vi "JTAG Panel.vi"() -> ()   [LabVIEW 2009]
panel:
  in  "Function":u16(ring) items=["READ_IO_VARS"=0, "PORT_OUT"=1, "PORT_SEL"=2, "PORT_REN"=3, "PORT_IN"=4, "PORT_DIR"=5, "SET_LCM"=6, "PWR_WRITE_SINGLE"=12, "PWR_READ_SINGLE"=13, "PWR_WRITE_MASK"=16, "PWR_WRITE_TRIM_DEFAULTS"=17, "STIM_POWER_UP"=20, "STIM_POWER_DN"=21, "STIM_WRITE_SINGLE"=22, "STIM_READ_SINGLE"=23, "STIM_WRITE_BLOCK"=24, "STIM_READ_BLOCK"=25, "STIM_WRITE_MASK"=26, "MICS_POWER_UP"=30, "MICS_POWER_DN"=31, "MICS_WRITE_SINGLE"=32, "MICS_READ_SINGLE"=33, "MICS_WRITE_BLOCK"=34, "MICS_READ_BLOCK"=35, "MICS_WRITE_MASK"=36, "MEM_POWER_UP"=40, "MEM_POWER_DN"=41, "MEM_WRITE_SINGLE"=42, "MEM_READ_SINGLE"=43, "MEM_WRITE_BLOCK"=44, "MEM_READ_BLOCK"=45, "MEM_WRITE_MASK"=46, "MEM_WRITE_SR"=47, "MEM_READ_SR"=48, "MEM_WRITE_OPCODE"=49, "INIT_PORTS"=50, "INIT_COMMS"=60, "RELEASE_COMMS"=61, "INIT_VARS"=62, "DCO_1MHZ"=63, "DCO_8MHZ"=64, "STANDARD_STARTUP"=65, "SET_LCM"=66, "PLUTO_WRITE_TRIM_DEFAULTS"=67, "SATURN_DIG_STARTUP"=68, "SATURN_BBC_STARTUP"=69, "SATURN_BBC_SHUTDOWN"=70, "START_STIM_CLK"=80, "STOP_STIM_CLK"=81, "PULSE_STIM_CLK"=82, "PULSE_STIM_SCK"=83, "SINGLE_ADC12"=85, "SINGLE_ADC12_REPEAT"=86, "MULTI_ADC12"=87, "MULTI_ADC12_REPEAT"=88, "DISABLE_ADC12"=89, "TC_STIM_RAM_READ"=200, "TC_STIM_RAM_WRITE"=201, "TC_TIMING_TEST"=220]
  out "error out":errorcluster
  out "MD5 message-digest out":string
  out "Status":bool
  in  "MD5 message-digest in":string
  in  "Function":T1(ring)
  in  "File Path":path=path "C:/Documents and Settings/Operator/My Documents/workspace_2/Test_Firmware_V1/Release/Test_Firmware_V1.txt"
  in  "Do Program":bool
  out "error out 3":errorcluster
  out "ARG1-ARG7":u16[](array[numeric]) format="%04x"
  out "ARG 7":u16 format="%04x"
  in  "ARG 6":u16 format="%04x"
  in  "ARG 5":u16 format="%04x"
  in  "ARG 4":u16 format="%04x"
  in  "ARG 3":u16 format="%04x"
  in  "ARG 2":u16 format="%04x"
  in  "ARG 1":u16 format="%04x"
  in  "Quick Bit Function (Manual)":T2(ring)
  in  "Function":u16(ring)=3 items=["Power UP", "Power DN", "Write Single", "Read Single", "Write Block", "Read Block", "Write Masked", "Test Value"]
  in  "State (L)":bool
  in  "RESET TARGET":bool
  in  "START MCU ZERO":bool
  in  "START MCU":bool
  in  "Sync JTAG (STOP MCU)":bool
  out "Device Vcc":dbl
  out "error out":errorcluster
  out "Block Read Data":u16[](array[numeric]) format="%02x"
  out "Test Result":bool
  out "Read Value":u8 format="%02x"
  in  "Block Write Data":u8[](array[numeric]) format="%02x"
  in  "Blocksize":u16
  in  "Target":u16(ring) items=["Power ASIC", "Stim ASIC", "MICS Radio", "FRAM"]
  in  "Address":u16 format="%04x"
  in  "Value":u8 format="%02x"
  in  "Mask":u8 format="%02x"
  in  "SPI":bool
  in  "Buffer Address (Byte from Buffer)":u16=4352 format="%x"
  out "Byte OUT (Byte from Buffer)":u8 format="%x"
  in  "Byte from Buffer":bool
  in  "Buffer Address (Byte to Buffer)":u16=4352 format="%x"
  in  "Byte IN (Byte to Buffer)":u8
  in  "Byte to Buffer":bool
  in  "Block size (Buffer to RAM)":u16=18 format="%x"
  in  "Start address (Buffer to RAM)":u16=4352 format="%x"
  in  "Buffer to RAM":bool
  in  "Block size (RAM to Buffer)":u16=18 format="%x"
  in  "Start address (RAM to Buffer)":u16=4352 format="%x"
  in  "RAM to Buffer":bool
  in  "Power Target Device (Init)":bool=TRUE
  in  "Initialize":bool
  in  "Power Target Device (Release)":bool
  in  "Release":bool
  in  "Function":u16(ring)=5 items=["Initialize COMMs", "Release COMMs", "Initialize Variables", "Select 1MHz DCO", "Select 8MHz DCO", "Standard Startup"]
  in  "Config":bool
  in  "stop":bool
  in  "Function":T3(ring)
  out "error out 2":errorcluster
  out "Manual Read":u8 format="%02x"
  out "Quick Bit Read":bool
  in  "Mask (0)":u8 format="%02x"
  in  "Value (0)":u8 format="%02x"
  in  "Port (1)":T4(ring)
  in  "DO STATE":bool
  in  "Do BASE FUNCTION":bool
  # "Manual Inputs"
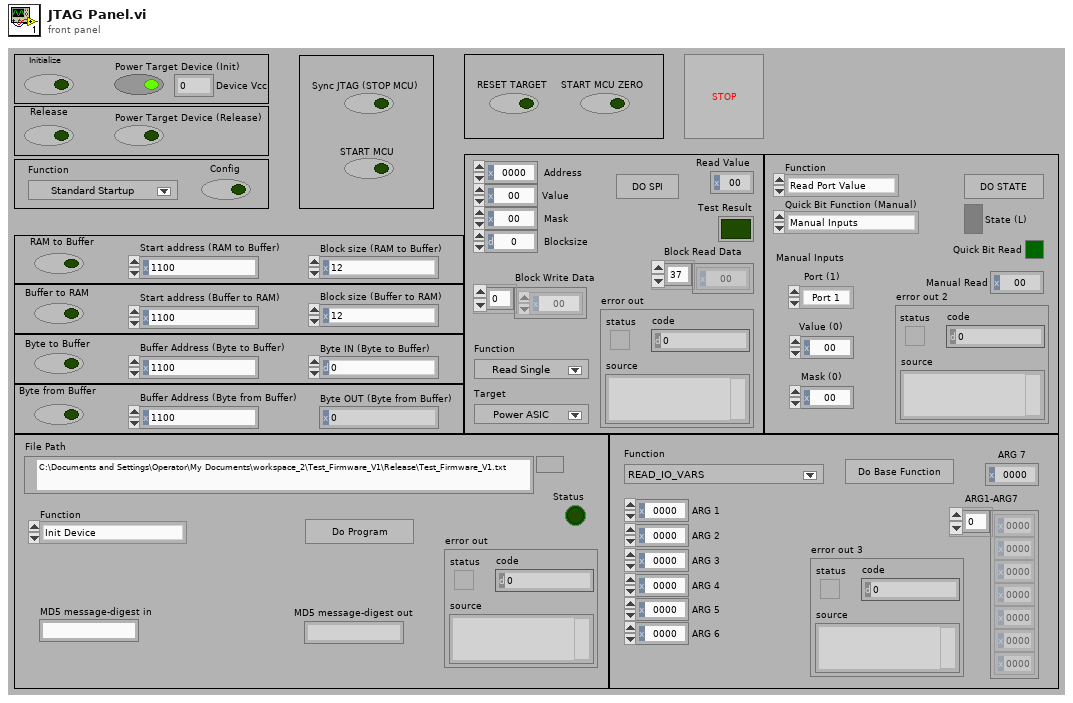
[diagram p1: front panel]
types:
  T1 = enum16{"Init Device", "Auto-Program from File", "Load New Code File", "Close Device", "Blank Check Device", "Erase Device Flash", "Program File to Flash", "Verify Flash vs File", "Read Flash to File", "Checksum of File", "Compare Checksums"}
  T2 = enum16{"Manual Inputs", "PWR_LDO_EN", "PWR_STROBE_IN", "PWR_UV_PROT", "PWR_MAG_TO_OVRD", "PWR_BBC_CTL", "PWR_HVDD_CONN", "<Reserved_1>", "<Reserved_2>", "STIM_RUN", "STIM_STOP", "STIM_CONT", "STIM_SEL", "RST_N", "<Reserved_3>", "TETS_TXD", "<Reserved_4>", "<Reserved_5>", "PWR_MAG_SW (IN)", "PWR_MAG_2S (IN)", "PWR_MAG_5S (IN)", "TETS_RXD (IN)", "PWR_V_DET (IN)", "PWR_BRWN_OUT (IN)", "MICS_IRQ", "<Reserved_7>", "STIM_PROG (IN)", "STIM_PAUSE (IN)", "STIM_SYNC (IN)", "STIM_TFLG (IN)", "STIM_ERR (IN)"}
  T3 = enum16{"Read Port Value", "Set Port Value", "Set Port Direction", "Set Port Select", "Set Port Res En"}
  T4 = enum8{"Port 1", "Port 2", "Port 3", "Port 4", "Port 5", "Port 6", "Port 7", "Port 8"}
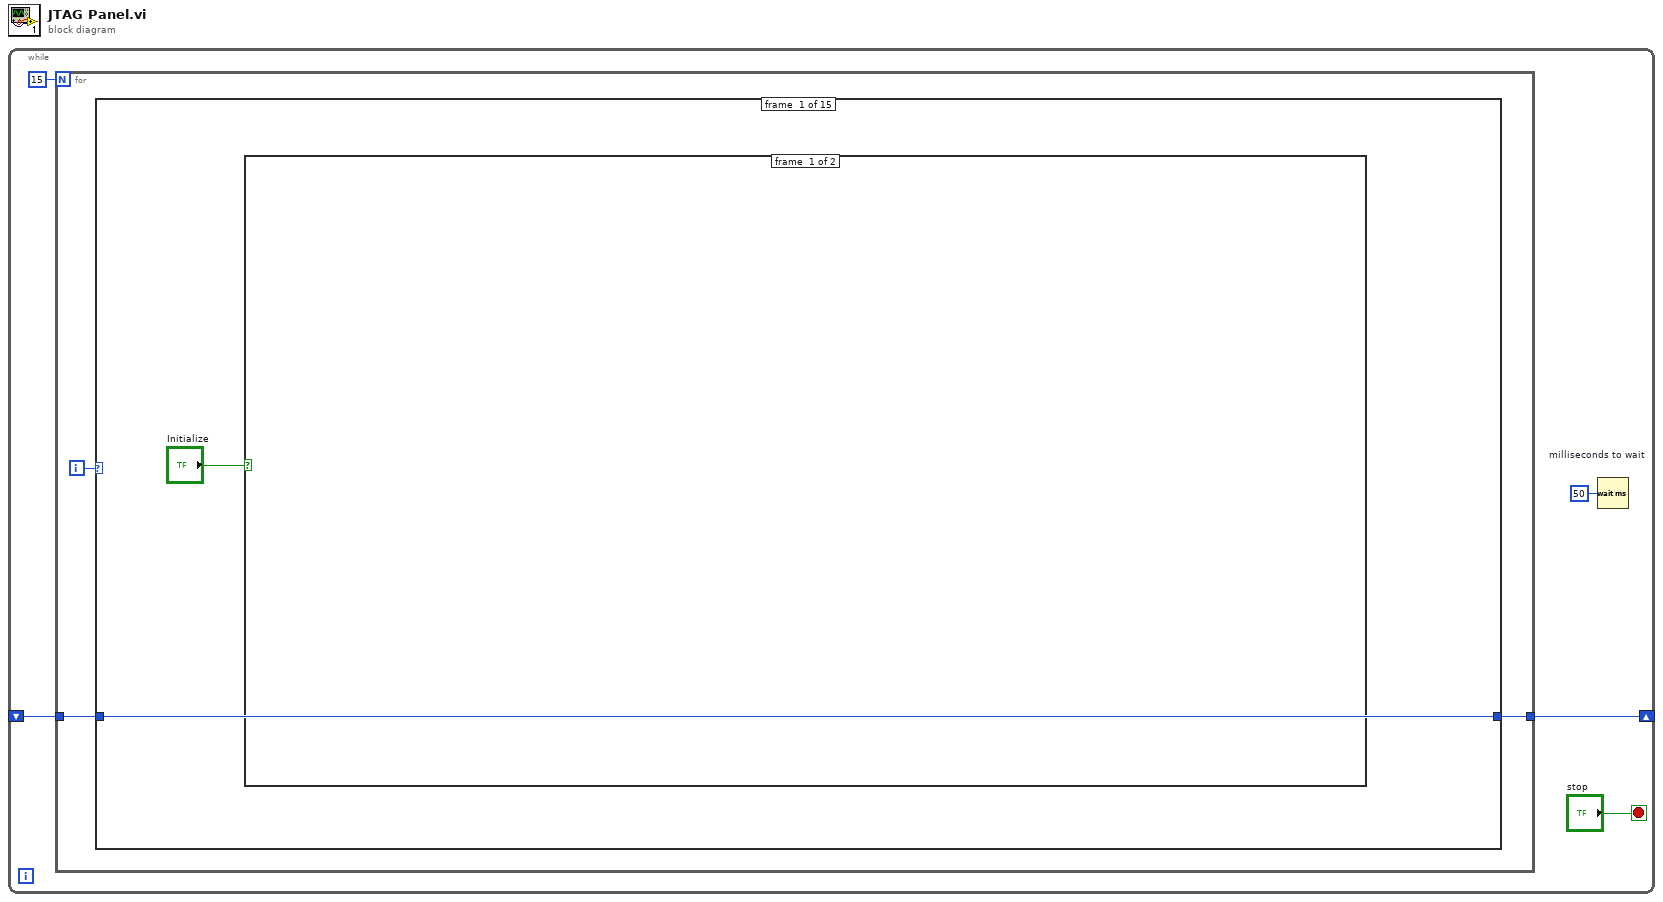
[diagram p0: block diagram]
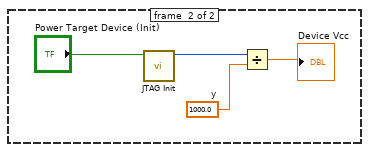
[diagram p2: hidden frame]
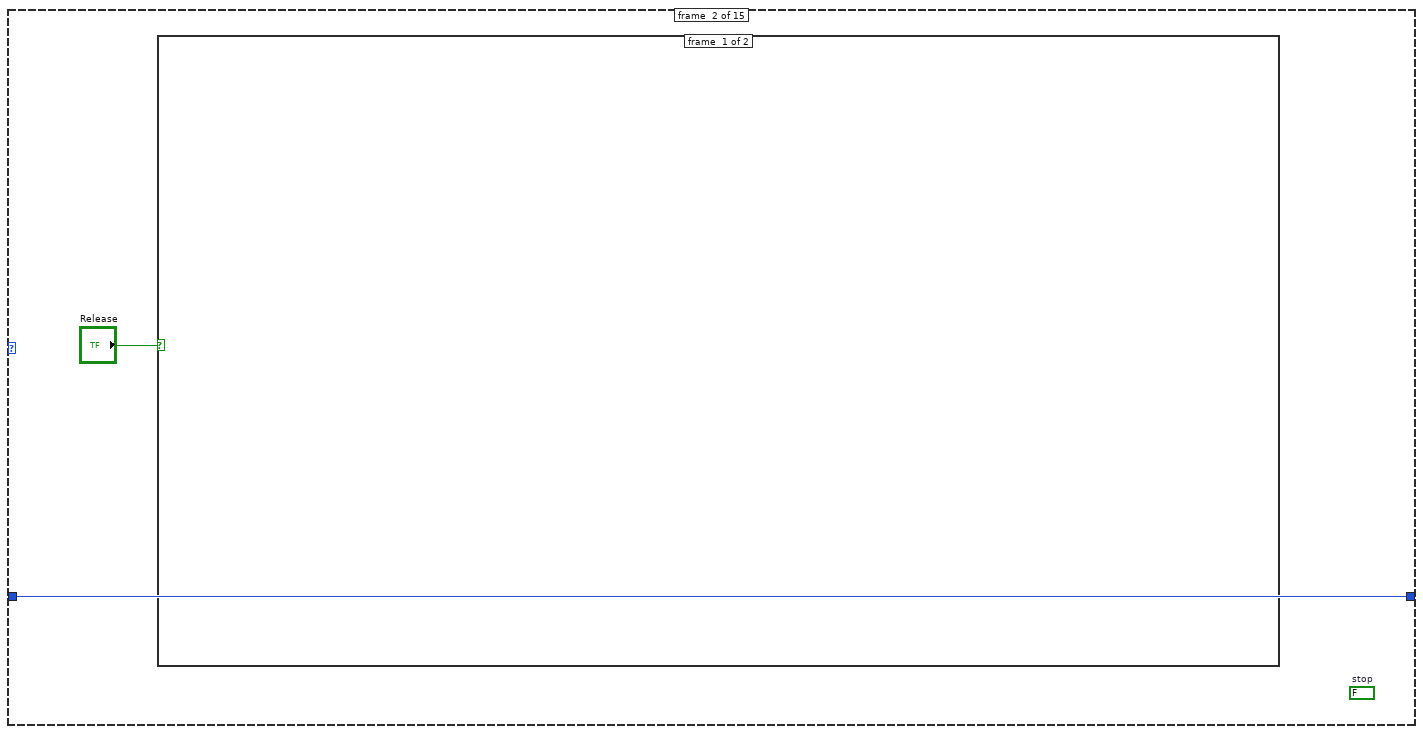
[diagram p3: hidden frame]
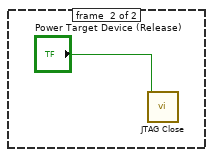
[diagram p4: hidden frame]
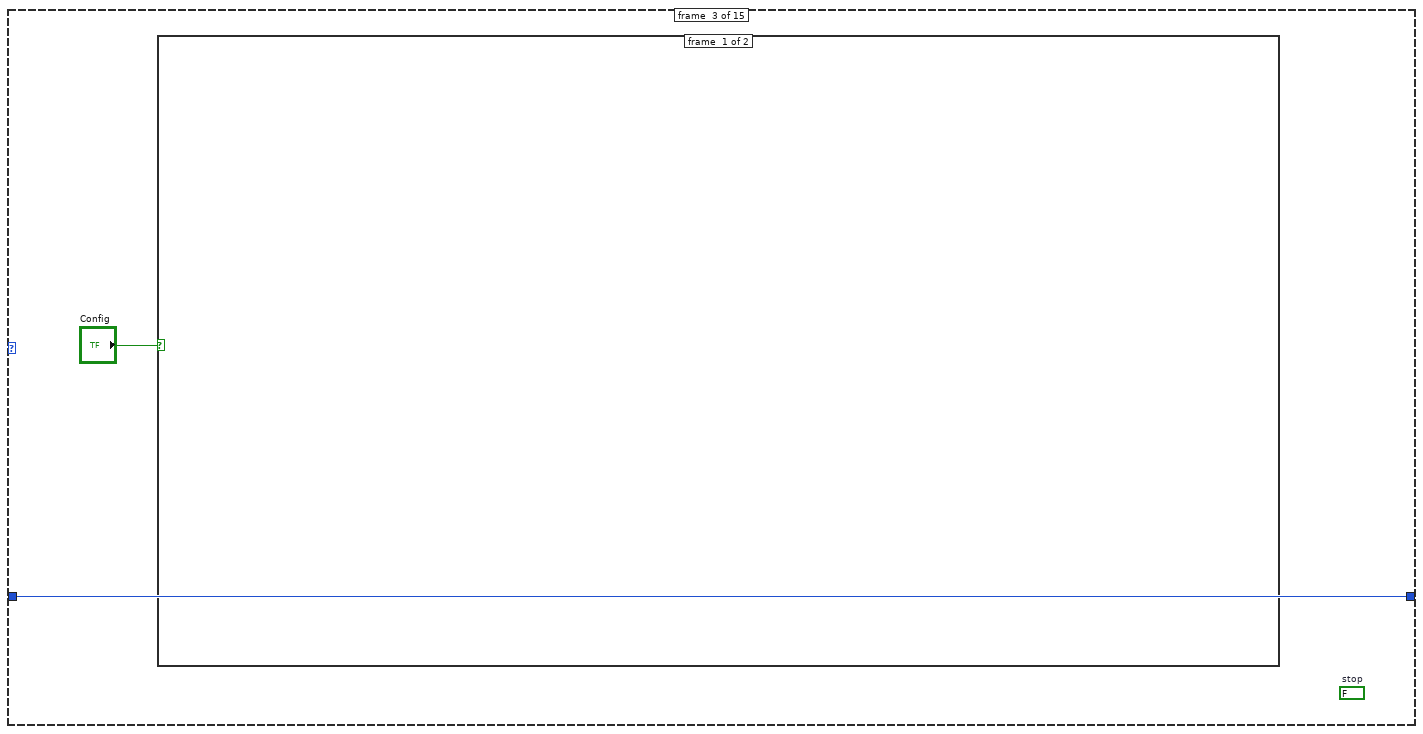
[diagram p5: hidden frame]
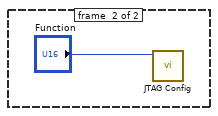
[diagram p6: hidden frame]
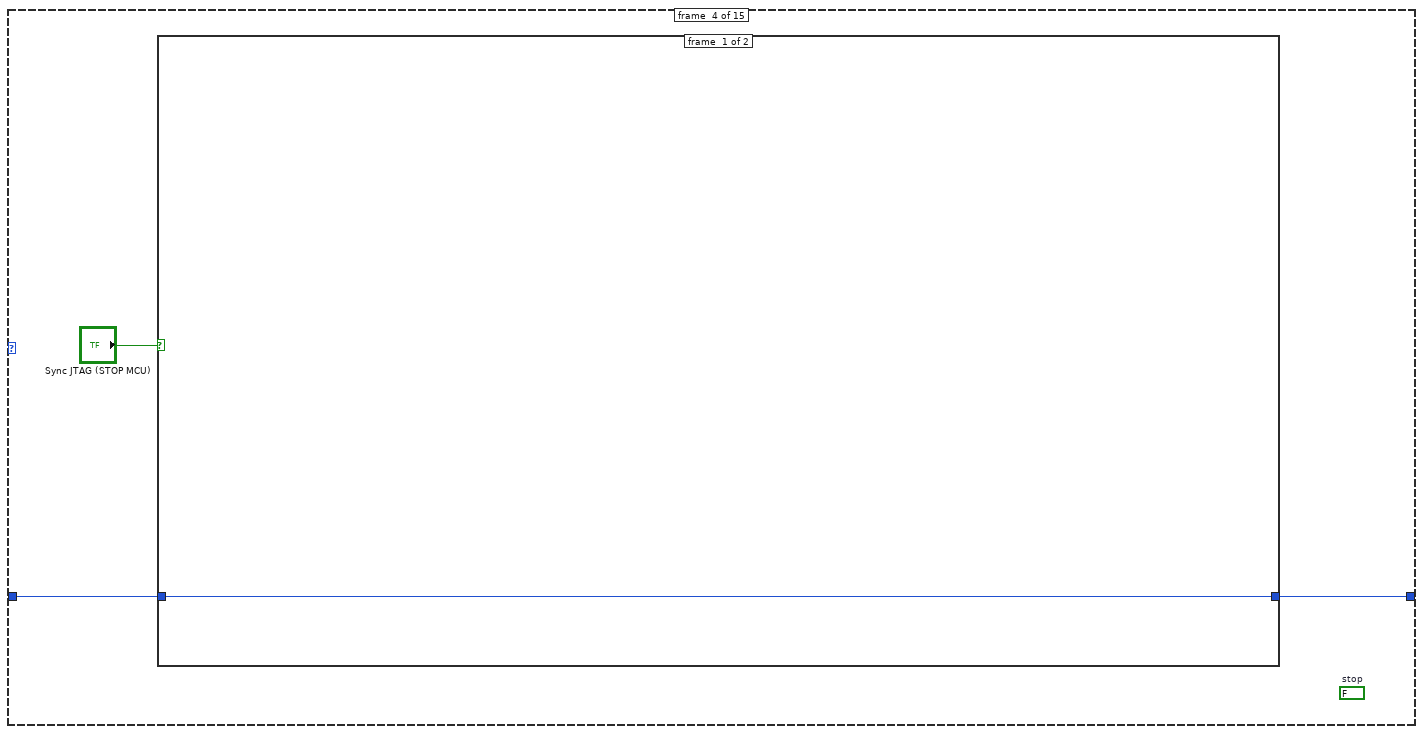
[diagram p7: hidden frame]
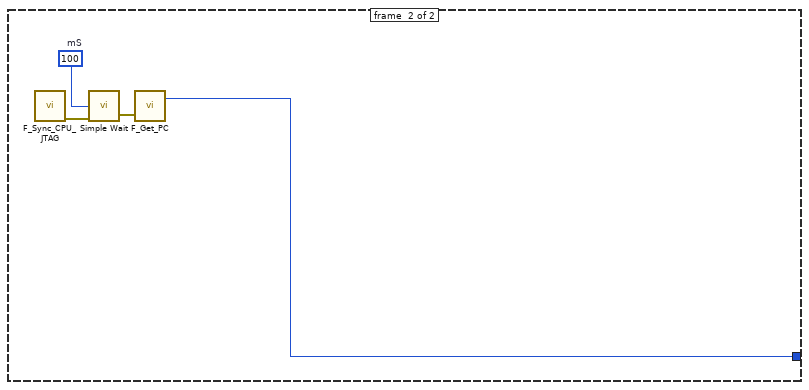
[diagram p8: hidden frame]
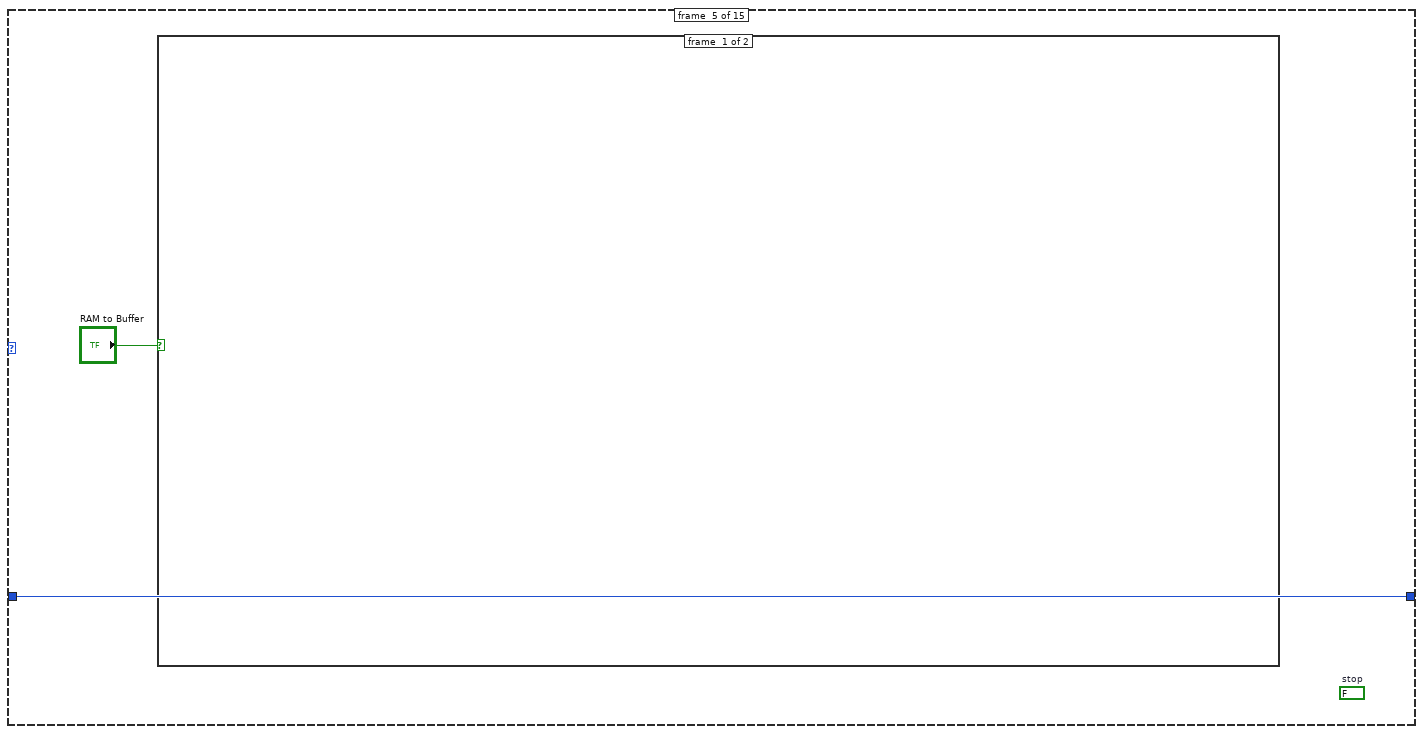
[diagram p9: hidden frame]
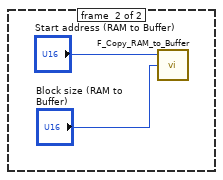
[diagram p10: hidden frame]
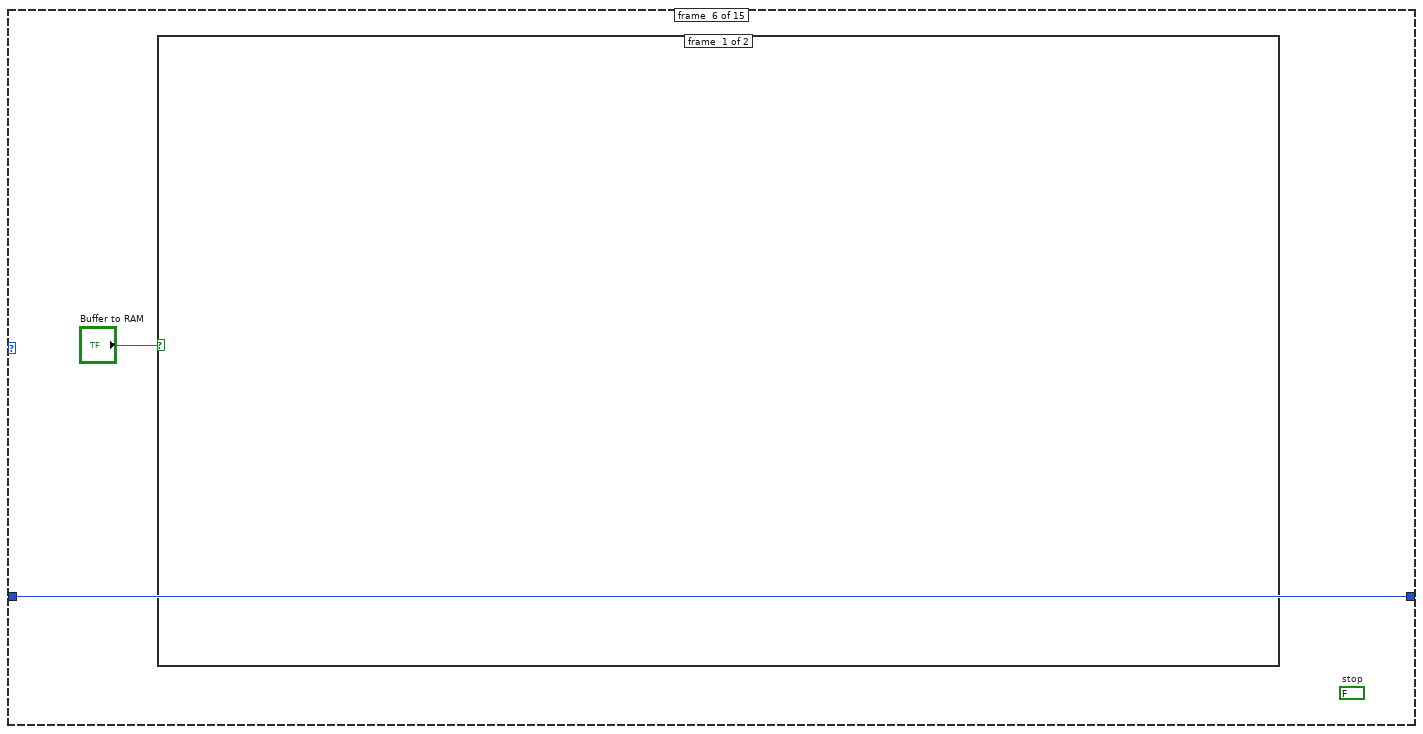
[diagram p11: hidden frame]
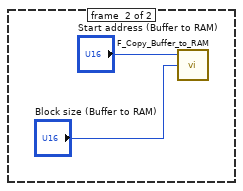
[diagram p12: hidden frame]
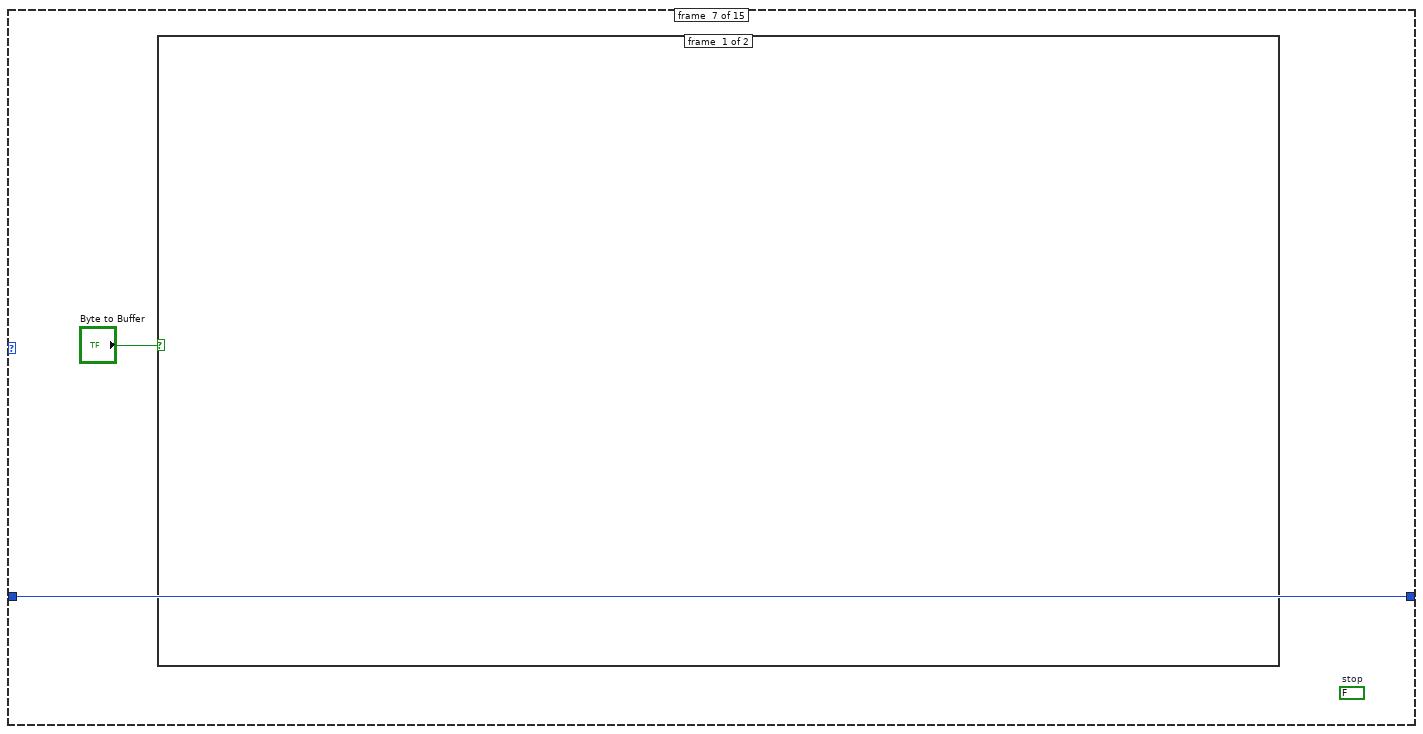
[diagram p13: hidden frame]
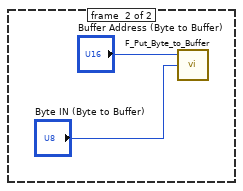
[diagram p14: hidden frame]
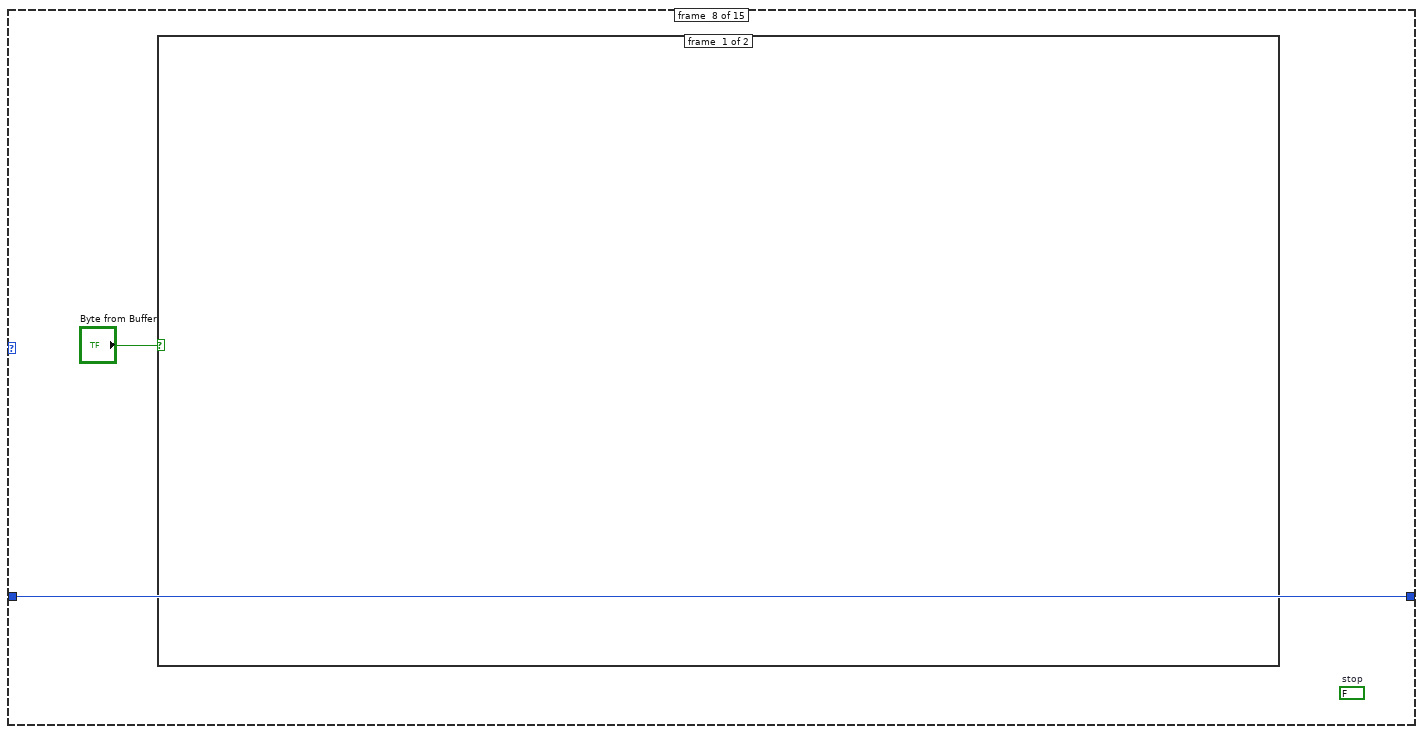
[diagram p15: hidden frame]
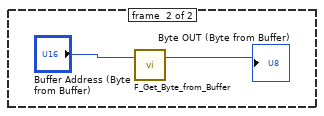
[diagram p16: hidden frame]
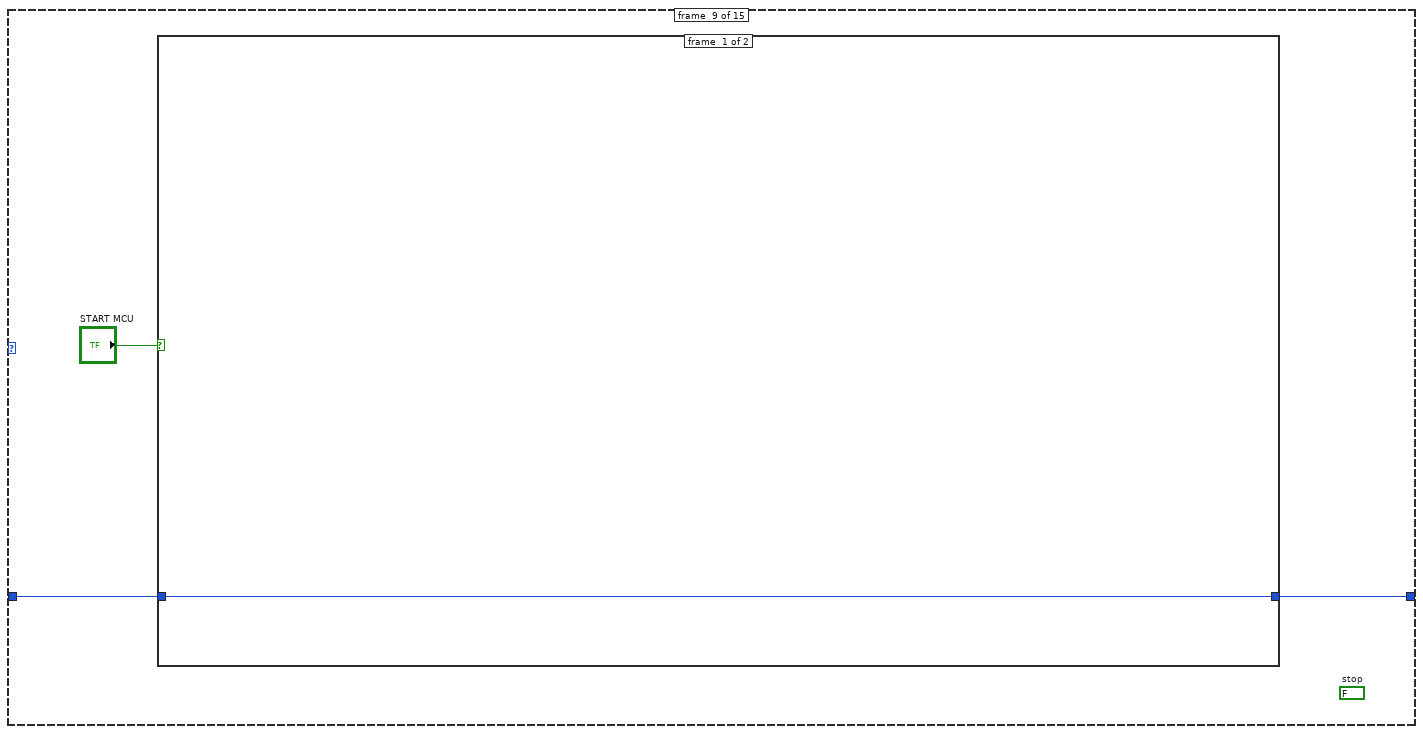
[diagram p17: hidden frame]
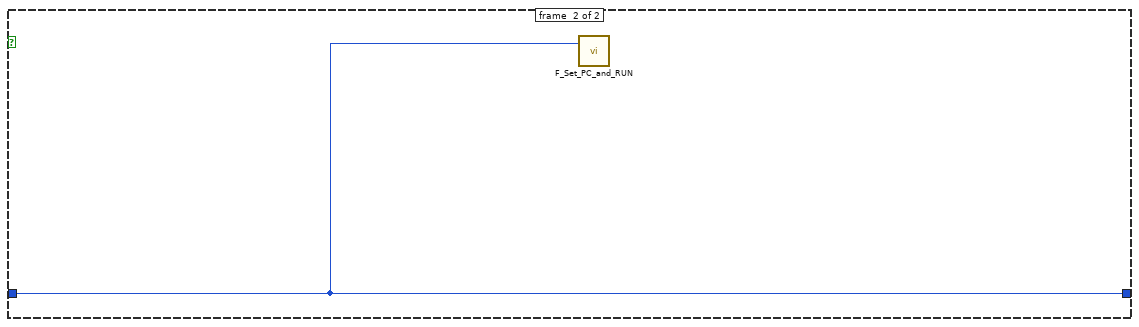
[diagram p18: hidden frame]
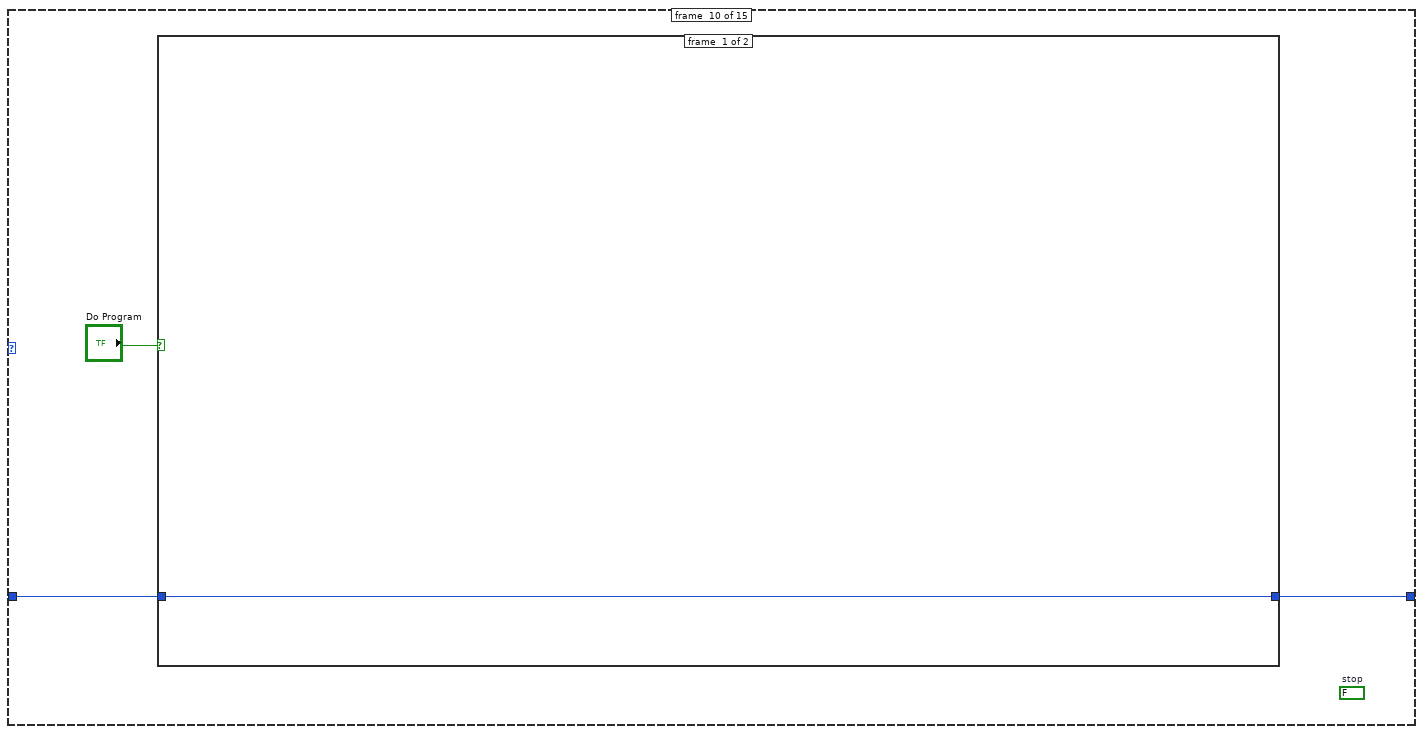
[diagram p19: hidden frame]
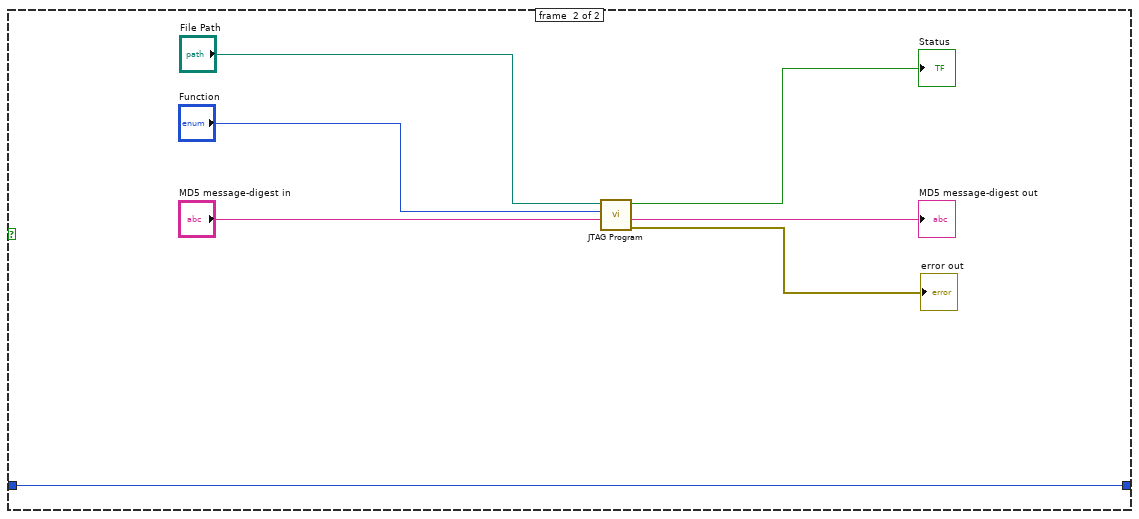
[diagram p20: hidden frame]
diagram:
  n1 = while {
    shift-right: [w4] -> _
    shift-left: _ -> [w3]
    stop <- "stop" stop-if-true
    w1 = u32 50  # milliseconds to wait
    n2 = for {
      N: 15 -> [_]
      tunnel: [w7] -> w4
      tunnel: w3 -> [w6]
      i -> [w8]
      n3 = case shown="13" w8 {
        tunnel: [w9 w15 w18 w22 w29 w33 w37 w41 w45 w51 w61 w75 w81 w85 w99] -> w7
        tunnel: w6 -> [w9 w15 w18 w21 w29 w33 w37 w41 w46 w52 w62 w76 w80 w85 w99]
        frame #0 {
          n4 = case shown="True" "Initialize" {
            frame #0 {
            }
            frame #1 {
              w12 = 1000.0  # y
              n5 = call "JTAG Init.vi"("Power Target Device"="Power Target Device (Init)") -> ("Device Vcc"=w11:i32)  [unwired: 9 in, 1 out]
              n6 = Divide(x=w11, y=w12) -> (x/y=→"Device Vcc":dbl)
            }
          }
        }
        frame #1 {
          (unwired) FALSE  # stop
          n7 = case shown="True" "Release" {
            frame #0 {
            }
            frame #1 {
              n8 = call "JTAG Close.vi"("Power Target Device"="Power Target Device (Release)") -> ()  [unwired: 10 in, 1 out]
            }
          }
        }
        frame #2 {
          (unwired) FALSE  # stop
          n9 = case shown="True" "Config" {
            frame #0 {
            }
            frame #1 {
              n10 = call "JTAG Config.vi"("Function"="Function") -> ()  [unwired: 10 in, 1 out]
            }
          }
        }
        frame #3 {
          (unwired) FALSE  # stop
          n11 = case shown="True" "Sync JTAG (STOP MCU)" {
            tunnel: [w24 w25] -> w22
            tunnel: w21 -> [w24 _]
            frame #0 {
            }
            frame #1 {
              w26 = u32 100  # mS
              n12 = call "F_Sync_CPU_JTAG.vi"() -> ("error out"=w27:errorcluster)  [unwired: 2 in, 1 out]
              n13 = call "Simple Wait.vi"("mS"=w26, "error in"=w27) -> ("error out"=w28:errorcluster)  [unwired: 12 in, 1 out]
              n14 = call "F_Get_PC.vi"("error in (no error)"=w28) -> ("Program Counter"=w25:u16)  [unwired: 1 in, 1 out]
            }
          }
        }
        frame #4 {
          (unwired) FALSE  # stop
          n15 = case shown="True" "RAM to Buffer" {
            frame #0 {
            }
            frame #1 {
              n16 = call "F_Copy_RAM_to_Buffer.vi"("Block size to be copied"="Block size (RAM to Buffer)", "RAM start address"="Start address (RAM to Buffer)") -> ()  [unwired: 3 in, 1 out]
            }
          }
        }
        frame #5 {
          (unwired) FALSE  # stop
          n17 = case shown="True" "Buffer to RAM" {
            frame #0 {
            }
            frame #1 {
              n18 = call "F_Copy_Buffer_to_RAM.vi"("Block size to be copied"="Block size (Buffer to RAM)", "Buffer start address"="Start address (Buffer to RAM)") -> ()  [unwired: 3 in, 1 out]
            }
          }
        }
        frame #6 {
          (unwired) FALSE  # stop
          n19 = case shown="True" "Byte to Buffer" {
            frame #0 {
            }
            frame #1 {
              n20 = call "F_Put_Byte_to_Buffer.vi"("New value"="Byte IN (Byte to Buffer)", "Address of byte to be updated"="Buffer Address (Byte to Buffer)") -> ()  [unwired: 3 in, 1 out]
            }
          }
        }
        frame #7 {
          (unwired) FALSE  # stop
          n21 = case shown="True" "Byte from Buffer" {
            frame #0 {
            }
            frame #1 {
              n22 = call "F_Get_Byte_from_Buffer.vi"("Address of byte to be read"="Buffer Address (Byte from Buffer)") -> ("Current value"=→"Byte OUT (Byte from Buffer)":u8)  [unwired: 1 in, 1 out]
            }
          }
        }
        frame #8 {
          (unwired) FALSE  # stop
          n23 = case shown="True" "START MCU" {
            tunnel: w46 -> [w48 w49]
            tunnel: [w48 w49] -> w45
            frame #0 {
            }
            frame #1 {
              n24 = call "F_Set_PC_and_RUN.vi"("PC start address"=w49) -> ()  [unwired: 2 in, 1 out]
            }
          }
        }
        frame #9 {
          (unwired) FALSE  # stop
          n25 = case shown="True" "Do Program" {
            tunnel: w52 -> [w53 w60]
            tunnel: [w53 w60] -> w51
            frame #0 {
            }
            frame #1 {
              n26 = call "JTAG Program.vi"("MD5 message-digest"="MD5 message-digest in", "Function"="Function", "File Path"="File Path") -> ("error out"=→"error out":errorcluster, "MD5 message-digest 2"=→"MD5 message-digest out":string, "Status"=→"Status":bool)  [unwired: 6 in]
            }
          }
        }
        frame #10 {
          (unwired) FALSE  # stop
          n27 = case shown="True" "DO STATE" {
            tunnel: w62 -> [w64 w74]
            tunnel: [w64 w74] -> w61
            frame #0 {
            }
            frame #1 {
              n28 = call "JTAG State.vi"("Quick Bit Function (Manual)"="Quick Bit Function (Manual)", "Port (1)"="Port (1)", "Value (0)"="Value (0)", "Mask (0)"="Mask (0)", "State (L)"="State (L)", "Function"="Function") -> ("Quick Bit Read"=→"Quick Bit Read":bool, "Manual Read"=→"Manual Read":u8, "error out"=→"error out 2":errorcluster)  [unwired: 7 in]
            }
          }
        }
        frame #11 {
          (unwired) FALSE  # stop
          n29 = case shown="True" "RESET TARGET" {
            tunnel: w76 -> [w78 _]
            tunnel: [w78 w79] -> w75
            frame #0 {
            }
            frame #1 {
              w79 = 12544  # PC start address
              n30 = call "F_Reset_Target.vi"() -> ()  [unwired: 1 in, 1 out]
            }
          }
        }
        frame #12 {
          (unwired) FALSE  # stop
          n31 = case shown="True" "START MCU ZERO" {
            tunnel: [w83 w84] -> w81
            tunnel: w80 -> [w83 _]
            frame #0 {
            }
            frame #1 {
              w84 = 12544  # PC start address
              n32 = call "F_Set_PC_and_RUN.vi"("PC start address"=w84) -> ()  [unwired: 2 in, 1 out]
            }
          }
        }
        frame #13 {
          n33 = case shown="True" "SPI" {
            frame #0 {
            }
            frame #1 {
              n34 = call "JTAG SPI.vi"("Block Write Data"="Block Write Data", "Mask"="Mask", "Blocksize"="Blocksize", "Value"="Value", "Target"="Target", "Function"="Function", "Address"="Address") -> ("error out"=→"error out":errorcluster, "Block Read Data"=→"Block Read Data":u16[], "Test Result"=→"Test Result":bool, "Read Value"=→"Read Value":u8)  [unwired: 1 in]
            }
          }
        }
        frame #14 {
          n35 = case shown="True" "Do BASE FUNCTION" {
            frame #0 {
            }
            frame #1 {
              n36 = call "JTAG Base Function.vi"("Function"="Function", "ARG 4"="ARG 4", "ARG 5"="ARG 5", "ARG 6"="ARG 6", "ARG 1"="ARG 1", "ARG 2"="ARG 2", "ARG 3"="ARG 3") -> ("ARG 7"=→"ARG 7":u16, "ARG1-ARG7"=→"ARG1-ARG7":u16[], "error out"=→"error out 3":errorcluster)  [unwired: 6 in]
            }
          }
        }
      }
    }
    n37 = Wait (ms)(milliseconds to wait=w1) -> ()  [unwired: 1 out]
  }
